vi "Error_subvi.vi"(0 "error in (no error)":errorcluster) -> (1 "status":bool, 2 "code":i32, 3 "source":string)   [LabVIEW 2020]
uses:
  <vilib>/Utility/error.llb/DialogType.ctl
panel:
  # "Handles the Error"
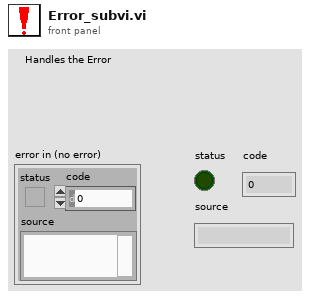
[diagram p1: front panel]
types:
  T1 = typedef "DialogType.ctl" = u16
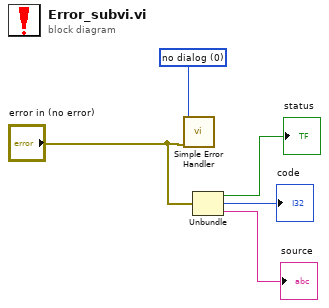
[diagram p0: block diagram]
diagram:
  w1 = T1 0 items=["no dialog", "OK message", "continue or stop message", "OK message + warnings", "continue/stop + warnings"] ("type of dialog (OK msg:1)")
  n1 = call <vilib>:"Simple Error Handler.vi"("type of dialog (OK msg:1)"=w1, "error in (no error)"="error in (no error)") -> ()  [unwired: 3 in, 5 out]
  n2 = Unbundle("error in (no error)") -> ("status"=→"status":bool, "code"=→"code":i32, "source"=→"source":string)
